vi "Test.vi"() -> ()   [LabVIEW 2019]
uses:
  Debug/KLInterface.dll
panel:
  in  "TestPoint":T1={"Position"={"Type"=enum."TEST_3", "Delay"=0.1, "CartesianPosition"={"X"=0.0, "Y"=0.0, "Z"=0.0, "ThetaX"=0.0, "ThetaY"=0.0, "ThetaZ"=0.0}, "Actuators"={"X"=0.0, "Y"=0.0, "Z"=0.0, "ThetaX"=0.0, "ThetaY"=0.0, "ThetaZ"=0.0}, "HandMode"=enum."TEST_3", "Fingers"={"Finger1"=0.0, "Finger2"=0.0, "Finger3"=0.0}}, "LimitationsActive"=FALSE, "SynchroType"=FALSE, "Limitations"={"speedParameter1"=0.0, "speedParameter2"=0.0, "speedParamerter3"=0.0, "forceParameter1"=0.0, "forceParameter2"=0.0, "forceParameter3"=0.0, "accelerationParameter1"=0.0, "accelerationParameter2"=0.0, "accelerationParameter3"=0.0}}
  out "return type":i32
  out "error out":errorcluster
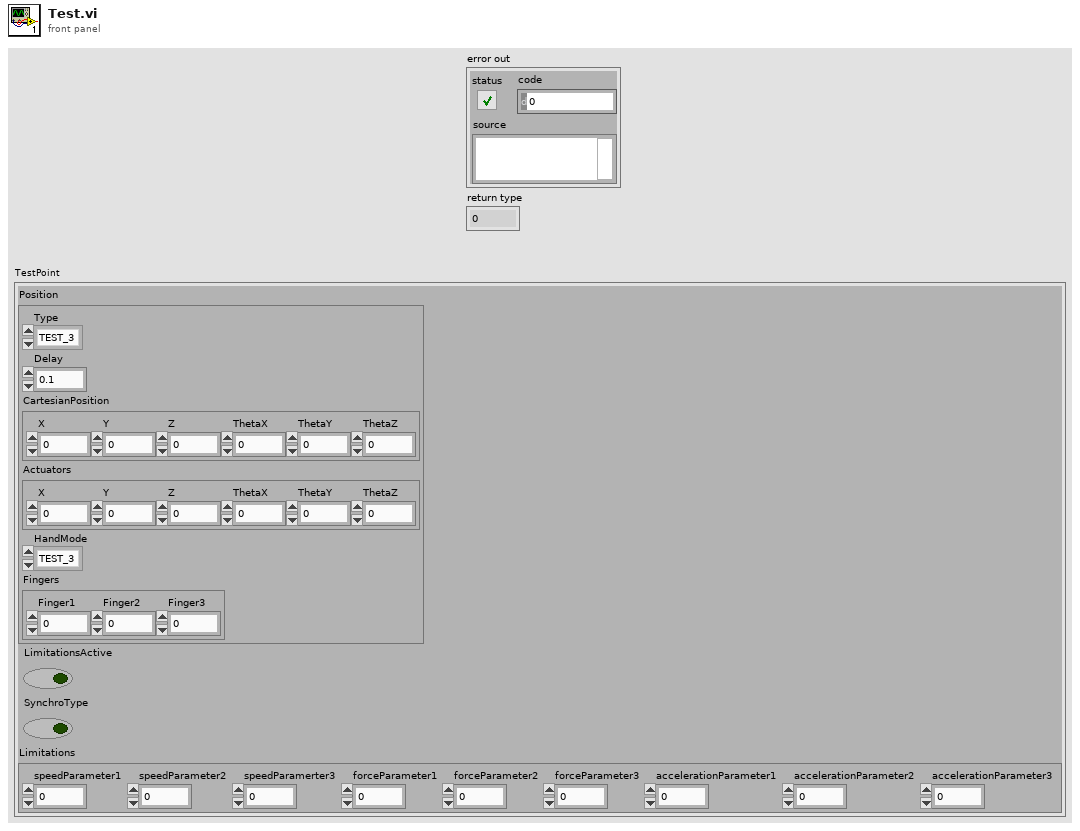
[diagram p1: front panel]
types:
  T1 = cluster{"Position":cluster{"Type":enum16{"TEST_3", "TEST_1", "TEST_2"}, "Delay":sgl, "CartesianPosition":cluster{"X":sgl, "Y":sgl, "Z":sgl, "ThetaX":sgl, "ThetaY":sgl, "ThetaZ":sgl}, "Actuators":cluster{"X":sgl, "Y":sgl, "Z":sgl, "ThetaX":sgl, "ThetaY":sgl, "ThetaZ":sgl}, "HandMode":enum16{"TEST_3", "TEST_1", "TEST_2"}, "Fingers":cluster{"Finger1":sgl, "Finger2":sgl, "Finger3":sgl}}, "LimitationsActive":bool, "SynchroType":bool, "Limitations":cluster{"speedParameter1":sgl, "speedParameter2":sgl, "speedParamerter3":sgl, "forceParameter1":sgl, "forceParameter2":sgl, "forceParameter3":sgl, "accelerationParameter1":sgl, "accelerationParameter2":sgl, "accelerationParameter3":sgl}}
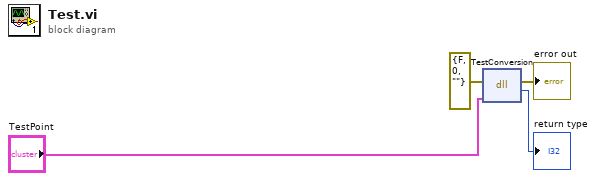
[diagram p0: block diagram]
diagram:
  n1 = dll-call lib="C:/Users/djcro/source/repos/ralphieraccoon/Kinova-Labview-Interface/Debug/KLInterface.dll" fn="TestConversion"(error in=errorcluster {"status"=FALSE, "code"=0, "source"=""} ("error in (no error)"), "test"="TestPoint") -> (error out=→"error out":errorcluster, "return type"=→"return type":i32)  [unwired: 3 in, 1 out]
